vi "Task Type.vi"(11 "Task in":refnum<class "Task.lvclass">) -> (2 "Task Type":string)   [LabVIEW 2020, in "Volatus.lvlib" / "Task.lvclass"]
uses:
  Task.lvclass
  Task.lvclass/Task.ctl
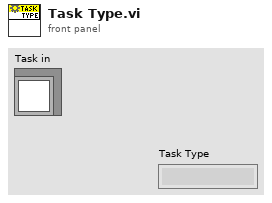
[diagram p1: front panel]
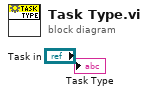
[diagram p0: block diagram]
diagram:
